vi "time conversion.vi"() -> ()   [LabVIEW 2018]
panel:
  out "time":dbl format="%<%H:%M:%S>t"
  in  "Numeric 2":dbl
  out "seconds":dbl
  out "minutes":dbl
  out "hours":dbl
  in  "Numeric":dbl
  # "170040320 - 9"
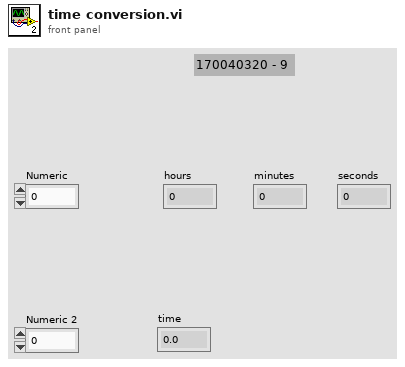
[diagram p1: front panel]
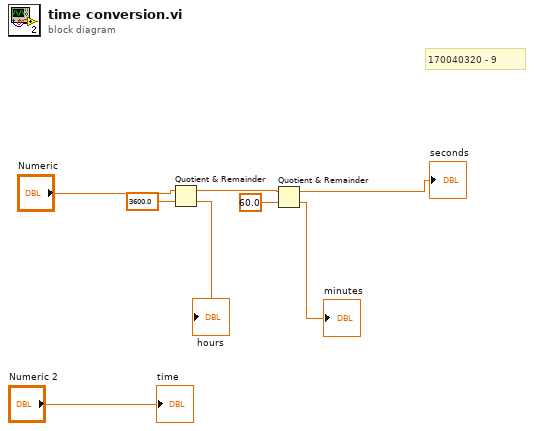
[diagram p0: block diagram]
diagram:
  # "170040320 - 9"
  n1 = Quotient & Remainder(x="Numeric", y=3600.0) -> (x-y*floor(x/y)=w5:dbl, floor(x/y)=→"hours":dbl)
  n2 = Quotient & Remainder(x=w5, y=60.0) -> (x-y*floor(x/y)=→"seconds":dbl, floor(x/y)=→"minutes":dbl)
  "time" <- "Numeric 2"
